vi "Reset Manual Layout.vi"(8 "error in":errorcluster, 11 "Manual UI in":refnum<class "Manual UI.lvclass">) -> (0 "error out":errorcluster, 3 "Manual UI out":refnum<class "Manual UI.lvclass">)   [LabVIEW 2023, in "Manual UI.lvlib" / "Manual UI.lvclass"]
uses:
  Project/Manual UI.lvclass
  Project/Manual UI.lvclass/Manual UI.ctl
  builds/Engine/Engine.lvlibp/Project/Engine.lvclass
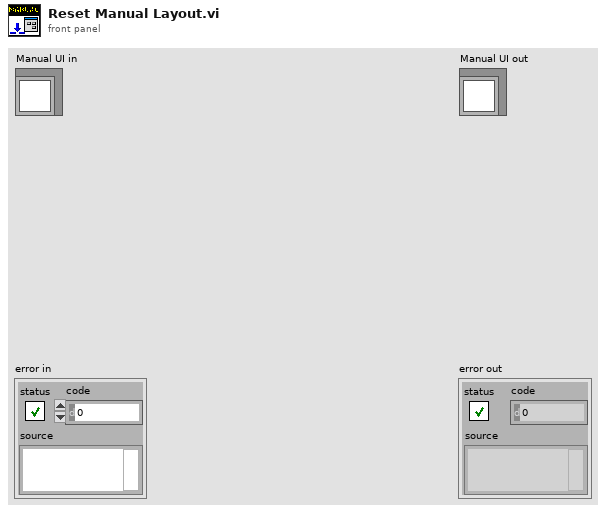
[diagram p1: front panel]
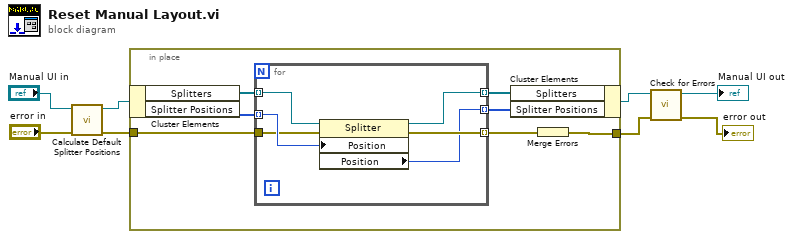
[diagram p0: block diagram]
diagram:
  n1 = call "Calculate Default Splitter Positions.vi"("error in"="error in", "Manual UI in"="Manual UI in") -> ("error out"=w2:errorcluster, "Manual UI out"=w1:refnum<class "Manual UI.lvclass">)  [unwired: 8 in]
  n2 = in-place {
    in-place-border: w2 -> [w13]
    in-place-border: [w11] -> w6
    n3 = in-place-cluster #1(w1) -> ("Splitters"=w15:refnum<vi>[], "Splitter Positions"=w10:i32[])
    n4 = for {
      tunnel: w15 -> [w21] mode=indexing
      tunnel: [w20] -> w14 mode=indexing
      tunnel: w13 -> [w17]
      tunnel: [w19] -> w12 mode=indexing
      tunnel: w10 -> [w18] mode=indexing
      tunnel: [w16] -> w9 mode=indexing
      n5 = property class="Splitter"(reference=w21, error in=w17, "Position"=w18) -> (reference out=w20:refnum<vi>, error out=w19:errorcluster, "Position"=w16:i32)
    }
    n6 = in-place-cluster #1("Splitters"=w14, "Splitter Positions"=w9) -> (w8:refnum<class "Manual UI.lvclass">)
    n7 = Merge Errors(w12) -> (w11:errorcluster)
  }
  n8 = call "Check for Errors.vi"("error in"=w6, "Engine in"=w8) -> ("error out"=→"error out":errorcluster, "Engine out"=→"Manual UI out":refnum<class "Manual UI.lvclass">)  [unwired: 8 in]
